vi "Arrange VIWin - Get Min Window Dimensions.vi"(0 "window type":T1, 11 "error in":errorcluster) -> (4 "min window dimensions":T2, 15 "error out":errorcluster)   [LabVIEW 2017, in "Arrange VI Window.lvlib"]
uses:
  Arrange VI Window.lvlib
  <resource>/dialog/lvconfig.llb/LV Config Read Numeric (I32).vi
  Arrange VIWin - Min Window Dimensions.ctl
  Arrange VIWin - Window Type.ctl
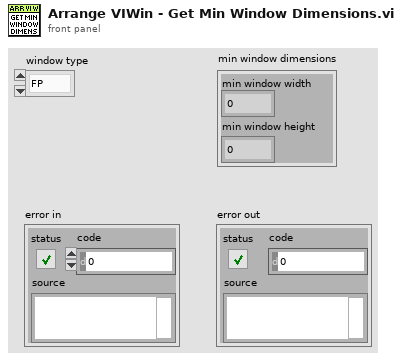
[diagram p1: front panel]
types:
  T1 = typedef "Arrange VI Window.lvlib/Arrange VIWin - Window Type.ctl" = enum16{"FP", "BD"}
  T2 = typedef "Arrange VI Window.lvlib/Arrange VIWin - Min Window Dimensions.ctl" = cluster{"min window width":i16, "min window height":i16}
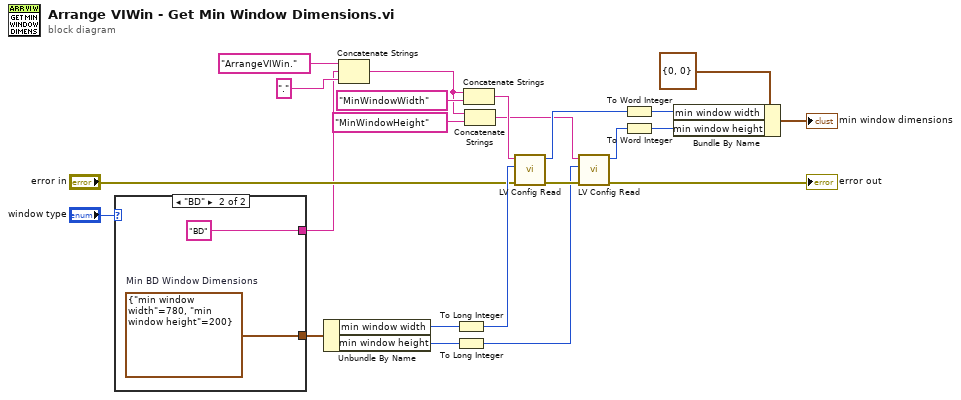
[diagram p0: block diagram]
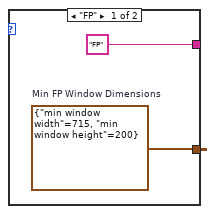
[diagram p2: hidden frame]
diagram:
  n1 = case shown="\"BD\"" "window type" {
    tunnel: [w24 w26] -> w11
    tunnel: ["FP" "BD"] -> w5
    frame "FP" {
      w24 = T2 {"min window width"=715, "min window height"=200}  # Min FP Window Dimensions
    }
    frame "BD" {
      w26 = T2 {"min window width"=780, "min window height"=200}  # Min BD Window Dimensions
    }
  }
  n2 = Unbundle By Name(w11) -> ("min window width"=w20:i16, "min window height"=w17:i16)
  n3 = Concatenate Strings("ArrangeVIWin." ("string"), w5, "." ("string")) -> (w2:string)
  n4 = To Long Integer(number=w20) -> (32bit integer=w19:i32)
  n5 = To Long Integer(number=w17) -> (32bit integer=w18:i32)
  n6 = Concatenate Strings(w2, "MinWindowWidth" ("key")) -> (w4:string)
  n7 = Concatenate Strings(w2, "MinWindowHeight" ("key")) -> (w1:string)
  n8 = call-poly <resource>:"LV Config Read.vi"("error in"="error in", "default value"=w19, "key"=w4) -> ("error out"=w22:errorcluster, "value"=w21:i32)  [unwired: 2 in, 1 out]
  n9 = call-poly <resource>:"LV Config Read.vi"("error in"=w22, "default value"=w18, "key"=w1) -> ("error out"=→"error out":errorcluster, "value"=w9:i32)  [unwired: 2 in, 1 out]
  n10 = To Word Integer(number=w21) -> (16bit integer=w15:i16)
  n11 = To Word Integer(number=w9) -> (16bit integer=w14:i16)
  n12 = Bundle By Name(cluster=T2 {"min window width"=0, "min window height"=0} ("Display:Primary Workspace"), "min window width"=w15, "min window height"=w14) -> (→"min window dimensions":T2)
